vi "Point to Waveform.vi"(6 "Channel name":string="Pump 1 Flow", 8 "error in (no error)":errorcluster, 9 "data":dbl=51.0, 10 "Time Stamp":timestamp=timestamp(3631881134.247515 s since 1904-01-01), 11 "dt":dbl=2000.0) -> (0 "error out":errorcluster, 3 "Waveform":waveform(dbl)={"t0"=timestamp(3631881134.247515 s since 1904-01-01), "dt"=2000.0, "Y"=[51.0], "attributes"=variant("NI_ChannelName"=variant(string "Pump 1 Flow"))})   [LabVIEW 2018, in "Waveform Loop.lvlib"]
uses:
  Waveform Loop.lvlib
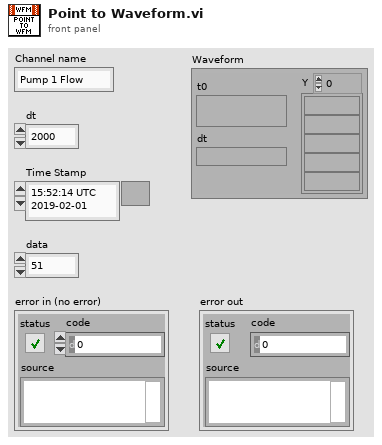
[diagram p1: front panel]
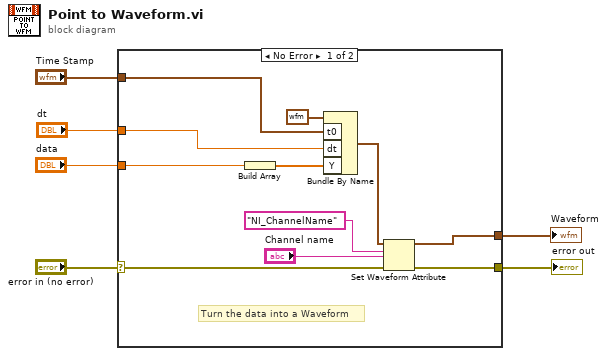
[diagram p0: block diagram]
diagram:
  n1 = case shown="No Error" "error in (no error)" {
    selector: "error in (no error)" -> [w7 w18]
    tunnel: [w17 _] -> w6
    tunnel: [w15 w18] -> w5
    tunnel: "data" -> [w12 _]
    tunnel: "dt" -> [w11 _]
    tunnel: "Time Stamp" -> [w10 _]
    frame No Error {
      # "Turn the data into a Waveform"
      n2 = Build Array(w12) -> (w13:dbl[])
      n3 = Bundle By Name(cluster=waveform(dbl) {"t0"=timestamp(0 s since 1904-01-01), "dt"=1.0, "Y"=[]} ("Waveform"), "t0"=w10, "dt"=w11, "Y"=w13) -> (w16:waveform(dbl))
      n4 = Set Waveform Attribute(4:w7, 5:"Channel name", 6:"NI_ChannelName" ("name"), 7:w16) -> (0:w15:errorcluster, 3:w17:waveform(dbl))  [unwired: 1 out]
    }
    frame Error {
    }
  }
  "Waveform" <- w6
  "error out" <- w5
